vi "mouse_to_image_coords.vi"(6 "Mouse Coords (screen/pane units)":cluster{"Left":dbl, "Top":dbl}, 7 "Image Control":refnum<vi>) -> (1 "Cursor is on Display Area":bool, 2 "Mouse Coords (image pixels)":cluster{dbl, dbl})   [LabVIEW 2019]
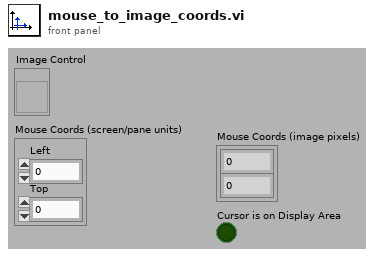
[diagram p1: front panel]
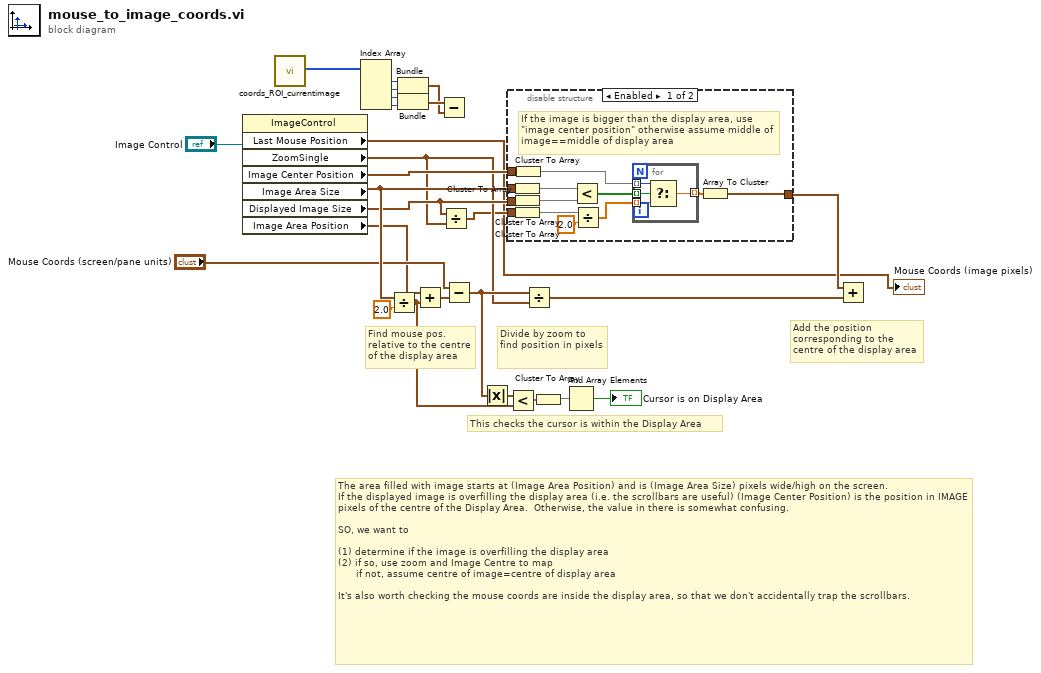
[diagram p0: block diagram]
diagram:
  # "This checks the cursor is within the Display Area"
  # "Add the position corresponding to the centre of the display area"
  # "Divide by zoom to find position in pixels"
  # "Find mouse pos. relative to the centre of the display area"
  # "The area filled with image starts at (Image Area Position) and is (Image Area Size) pixels wide/high on the screen.\nIf the displayed image is overfilling the display area (i.e. the scrollbars are useful) (Image Center Position) is the position in IMAGE pixels of the centre of the Display Area.  Otherwise, the value in there is somewhat confusing.\n\nSO, we want to \n\n(1) determine if the image is overfilling the display area\n(2) if so, use zoom and Image Centre to map\n      if not, assume centre of image=centre of display area\n\nIt's also worth checking the mouse coords are inside the display area, so that we don't accidentally trap the scrollbars."
  n1 = property class="ImageControl"(reference="Image Control") -> ("Last Mouse Position"=→"Mouse Coords (image pixels)":cluster{"X":i32, "Y":i32}, "ZoomSingle"=w3:cluster{"X":sgl, "Y":sgl}, "Image Center Position"=w25:cluster{"X":u32, "Y":u32}, "Image Area Size"=w23:cluster{"Width":u32, "Height":u32}, "Displayed Image Size"=w4:cluster{"Width":u32, "Height":u32}, "Image Area Position"=w6:cluster{"Left":i32, "Top":i32})  [unwired: 1 in, 2 out]
  n2 = call "coords_ROI_currentimage.vi"() -> ("Mono ROI"=w5:i32[])
  n3 = Index Array(array=w5) -> (element #1=w11:i32, element #2=w12:i32, element #3=w10:i32, element #4=w9:i32)  [unwired: 4 in]
  n4 = Divide(x=w23, y=2.0) -> (x/y=w16:cluster{"Width":dbl, "Height":dbl})
  n5 = Bundle("Numeric"=w11, "Numeric"=w12) -> (w7:cluster{"Numeric":i32, "Numeric":i32})  [unwired: 1 in]
  n6 = Bundle("Numeric"=w10, "Numeric"=w9) -> (w8:cluster{"Numeric":i32, "Numeric":i32})  [unwired: 1 in]
  n7 = Add(x=w6, y=w16) -> (x+y=w22:cluster{dbl, dbl})
  n8 = Subtract(x=w8, y=w7) -> ()  [unwired: 1 out]
  n9 = Divide(x=w4, y=w3) -> (x/y=w2:cluster{sgl, sgl})
  n10 = Subtract(x="Mouse Coords (screen/pane units)", y=w22) -> (x-y=w18:cluster{dbl, dbl})
  n11 = Absolute Value(x=w18) -> (abs(x)=w17:cluster{dbl, dbl})
  n12 = disable-structure shown="Enabled" {
    disable-tunnel: w23 -> [w31 _]
    disable-tunnel: w25 -> [w36 _]
    disable-tunnel: [w32 _] -> w19
    disable-tunnel: w2 -> [w30 _]
    disable-tunnel: w4 -> [w28 _]
    frame Enabled {
      # "If the image is bigger than the display area, use \"image center position\" otherwise assume middle of image==middle of display area"
      n13 = Cluster To Array(cluster=w31) -> (array=w35:u32[])
      n14 = Cluster To Array(cluster=w28) -> (array=w27:u32[])
      n15 = Cluster To Array(cluster=w30) -> (array=w29:sgl[])
      n16 = Cluster To Array(cluster=w36) -> (array=w34:u32[])
      n17 = Less?(x=w35, y=w27) -> (x < y?=w38:bool[])
      n18 = Divide(x=w29, y=2.0) -> (x/y=w37:dbl[])
      n19 = for {
        tunnel: w38 -> [w43] mode=indexing
        tunnel: w37 -> [w42] mode=indexing
        tunnel: w34 -> [w41] mode=indexing
        tunnel: [w40] -> w33 mode=indexing
        n20 = Select(t=w41, s=w43, f=w42) -> (s? t:f=w40:dbl)
      }
      n21 = Array To Cluster(array=w33) -> (cluster=w32:cluster{"[0]":dbl, "[1]":dbl})
    }
    frame Disabled {
    }
  }
  n22 = Less?(x=w17, y=w16) -> (x < y?=w15:cluster{bool, bool})
  n23 = Divide(x=w18, y=w3) -> (x/y=w20:cluster{dbl, dbl})
  n24 = Cluster To Array(cluster=w15) -> (array=w14:bool[])
  n25 = And Array Elements(Boolean array=w14) -> (logical AND=→"Cursor is on Display Area":bool)
  n26 = Add(x=w19, y=w20) -> ()  [unwired: 1 out]
